vi "deinitialize.vi"(0 "HGF_SVService":refnum<class "HGF_SVService.lvclass">, 5 "error in (no error)":errorcluster) -> (19 "error out":errorcluster)   [LabVIEW 2012, in "HGF_SV.lvlib" / "HGF_SVService.lvclass"]
doc: "This is a dynamic dispatch VI. It can be overwritten by childclasses to release allocated recources."
uses:
  HGF_SVService.lvclass
  HGF_BaseClasses/HGF_PVPublisher/HGF_PVPublisher.lvclass
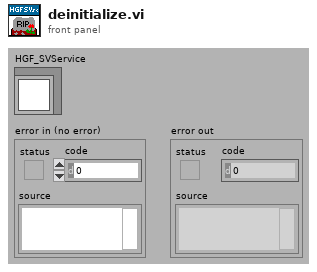
[diagram p1: front panel]
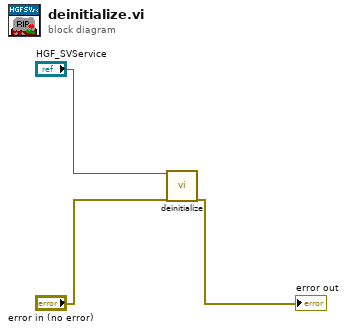
[diagram p0: block diagram]
diagram:
  n1 = call-parent "deinitialize.vi"("HGF_Factory"="HGF_SVService", "error in (no error)"="error in (no error)") -> ("error out"=→"error out":errorcluster)  [unwired: 17 out]
